vi "Get Background Image Relative Path.vi"(3 "Inkscape Path":path) -> (1 "Relative Path to Background":path)   [LabVIEW 2019]
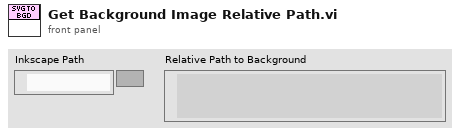
[diagram p1: front panel]
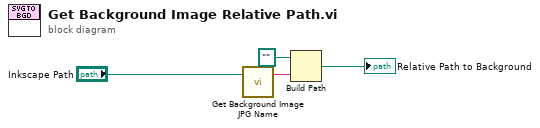
[diagram p0: block diagram]
diagram:
  n1 = call "Get Background Image JPG Name.vi"("Inkscape Path"="Inkscape Path") -> ("Background JPG Name"=w3:string)  [unwired: 2 in]
  n2 = Build Path(base path=path "", name or relative path=w3) -> (appended path=→"Relative Path to Background":path)
